vi "SetCurveLength.vi"(8 "error in (no error)":errorcluster caption="错误输入（无错误）", 11 "TPlot 输入":refnum<class "TPlot.lvclass">) -> (0 "error out":errorcluster caption="错误输出", 3 "TPlot 输出":refnum<class "TPlot.lvclass">)   [LabVIEW 2018, in "DataDisplay.lvlib" / "TPlot.lvclass"]
uses:
  TPlot.lvclass
  TPlot.lvclass/TPlot.ctl
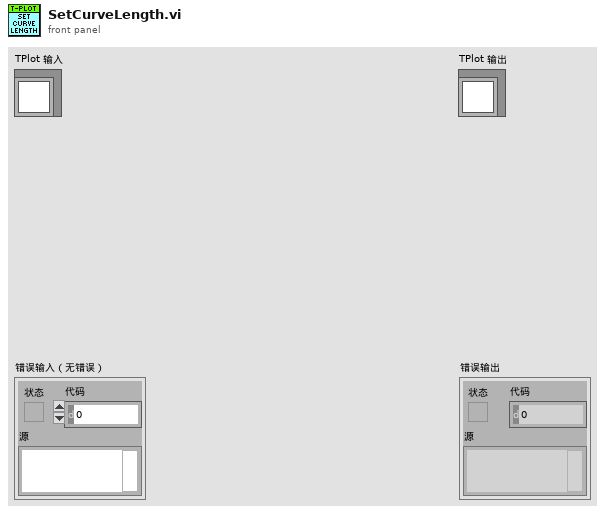
[diagram p1: front panel]
types:
  T1 = typedef "DataDisplay.lvlib/DD_CommandQ.ctl" = refnum<queue>
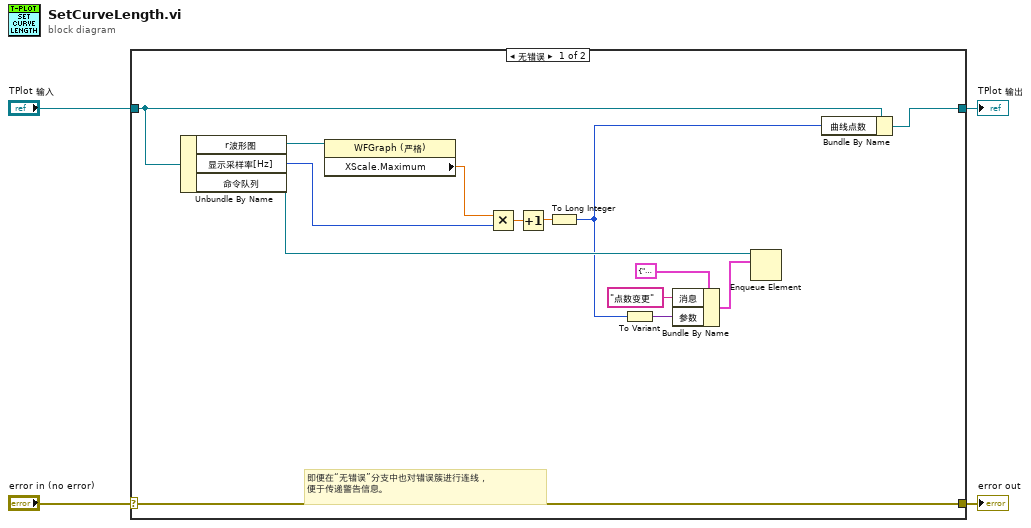
[diagram p0: block diagram]
diagram:
  n1 = case shown="无错误" "error in (no error)" {
    selector: "error in (no error)" -> [w18 w20]
    tunnel: [w18 w20] -> w3
    tunnel: [w11 w19] -> w1
    tunnel: "TPlot 输入" -> [w17 w19]
    frame No Error {
      # "即便在“无错误”分支中也对错误簇进行连线，\n便于传递警告信息。"
      n2 = Unbundle By Name(w17) -> ("r波形图"=w13:refnum<vi>, "显示采样率[Hz]"=w12:i32, "命令队列"=w10:T1)
      n3 = property class="WFGraph (严格)"(reference=w13) -> ("XScale.Maximum"=w16:dbl)  [unwired: 1 in, 2 out]
      n4 = Multiply(x=w16, y=w12) -> (x*y=w14:dbl)
      n5 = Increment(x=w14) -> (x+1=w15:dbl)
      n6 = To Long Integer(number=w15) -> (32bit integer=w5:i32)
      n7 = To Variant(anything=w5) -> (Variant=w6:variant)
      n8 = Bundle By Name(cluster=cluster{"消息":string, "参数":variant} {"消息"="", "参数"=variant} ("元素"), "消息"="点数变更", "参数"=w6) -> (w7:cluster{"消息":string, "参数":variant})
      n9 = Enqueue Element(queue=w10, element=w7) -> ()  [unwired: 2 in, 3 out]
      n10 = Bundle By Name(cluster=w17, "曲线点数"=w5) -> (w11:refnum<class "TPlot.lvclass">)
    }
    frame Error {
    }
  }
  "error out" <- w3
  "TPlot 输出" <- w1
